vi "PCO_GetMetaDataMode.vi"(8 "error in (no error)":errorcluster {"code" format="%x"}, 11 "ph":u64) -> (0 "error out":errorcluster {"code" format="%x"}, 1 "wMetaDataMode":u16(ring) items=["OFF", "ON"], 2 "ErrorMessage":i32 format="%x", 3 "ph out":u64, 4 "wMetaDataVersion":u16, 5 "wMetaDataSize":u16)   [LabVIEW 2019, in "SDK.lvlib" / "RecordingControl.lvlib"]
doc: "<b>Description:</b>\nThis function returns the current Meta Data mode of the camera and information about size and version of the Meta Data block.\nWhen Meta Data mode is enabled, a Meta Data block with additional information is added at the end of each image. The internal buffers allocated with PCO_AllocateBuffer are adapted automatically. If the buffers are allocated externally, further line(s) must be added, where the number of lines depends on horizontal resolution and the size of the additional Meta Data block.\n\n<b>Supported camera type:</b>\npco.dimax, pco.edge\n\n<b>Descriptor dependency:</b>\ndwGeneralCapsDESC1: METADATA"
uses:
  RecordingControl.lvlib
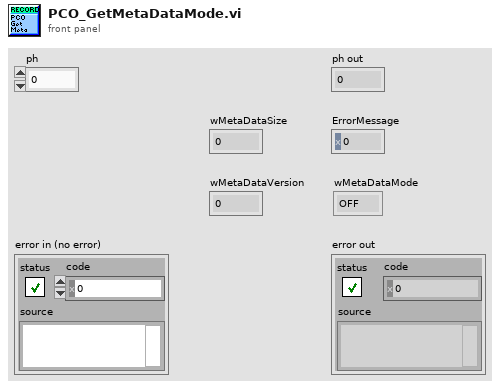
[diagram p1: front panel]
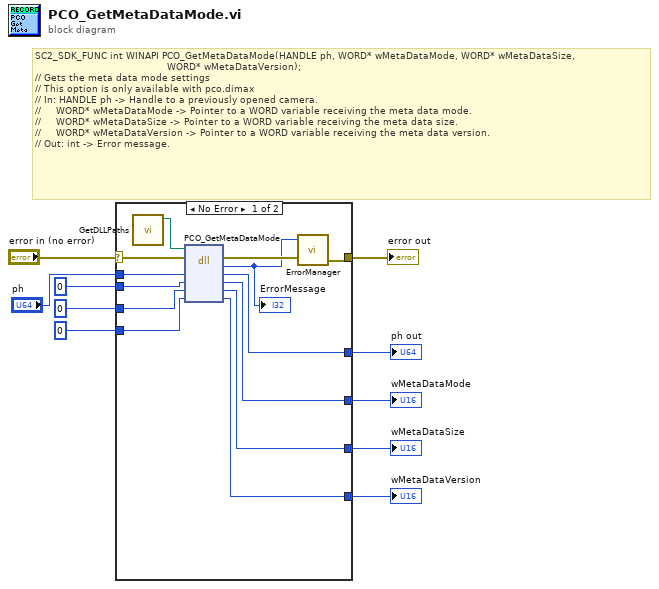
[diagram p0: block diagram]
diagram:
  # "SC2_SDK_FUNC int WINAPI PCO_GetMetaDataMode(HANDLE ph, WORD* wMetaDataMode, WORD* wMetaDataSize,\n                                            WORD* wMetaDataVersion);\n// Gets the meta data mode settings\n// This option is only available with pco.dimax\n// In: HANDLE ph -> Handle to a previously opened camera.\n//     WORD* wMetaDataMode -> Pointer to a WORD variable receiving the meta data mode.\n//     WORD* wMetaDataSize -> Pointer to a WORD variable receiving the meta data size.\n//     WORD* wMetaDataVersion -> Pointer to a WORD variable receiving the meta data version.\n// Out: int -> Error message."
  n1 = case shown="No Error" "error in (no error)" {
    selector: "error in (no error)" -> [w15 w28]
    tunnel: "ph" -> [w23 w27]
    tunnel: [w22 w27] -> w9
    tunnel: u16 0 ("wMetaDataMode") -> [w21 w26]
    tunnel: [w20 w26] -> w7
    tunnel: u16 0 ("wMetaDataSize") -> [w19 w25]
    tunnel: [w18 w25] -> w5
    tunnel: u16 0 ("wMetaDataVersion") -> [w17 w24]
    tunnel: [w16 w24] -> w3
    tunnel: [w13 w28] -> w2
    frame No Error {
      n2 = call "GetDLLPaths.vi"() -> ("SC2_Cam_Path"=w11:path)  [unwired: 9 in, 2 out]
      n3 = dll-call lib="?" fn="PCO_GetMetaDataMode"(path in=w11, error in=w15, "ph"=w23, "wMetaDataMode"=w21, "wMetaDataSize"=w19, "wMetaDataVersion"=w17) -> (error out=w14:errorcluster, "return type"=w12:i32, "ph"=w22:u64, "wMetaDataMode"=w20:u16, "wMetaDataSize"=w18:u16, "wMetaDataVersion"=w16:u16)  [unwired: 1 in, 1 out]
      "ErrorMessage" <- w12
      n4 = call "ErrorManager.vi"("error in (no error)"=w14, "error code"=w12) -> ("error out"=w13:errorcluster)  [unwired: 3 in]
    }
    frame Error {
    }
  }
  "ph out" <- w9
  "wMetaDataMode" <- w7
  "wMetaDataSize" <- w5
  "wMetaDataVersion" <- w3
  "error out" <- w2
